vi "TVS Test.vi"(8 "error in (no error)":errorcluster, 10 "Message IN":string) -> (0 "error out":errorcluster, 1 "Result (bool)":bool, 2 "Message OUT":string)   [LabVIEW 2022 SP3]
uses:
  <vilib>/DAQmx/write.llb/DAQmx Write (Digital Bool 1Line 1Point).vi
  <vilib>/DAQmx/read.llb/DAQmx Read (Digital Bool 1Line 1Point).vi
  <vilib>/DAQmx/miscellaneous.llb/DAQmx Fill In Error Info.vi
panel:
  out "DAQ Reading":bool
  out "Result (color)":u32(colorbox)
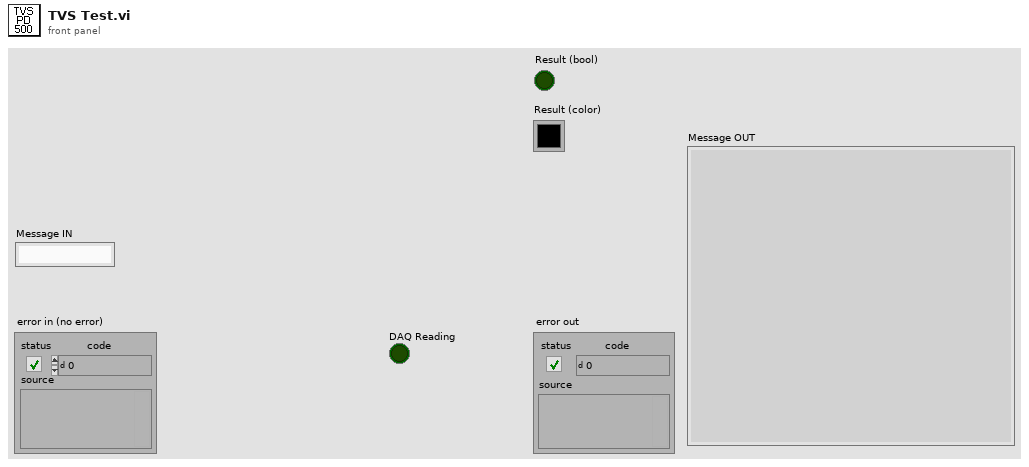
[diagram p1: front panel]
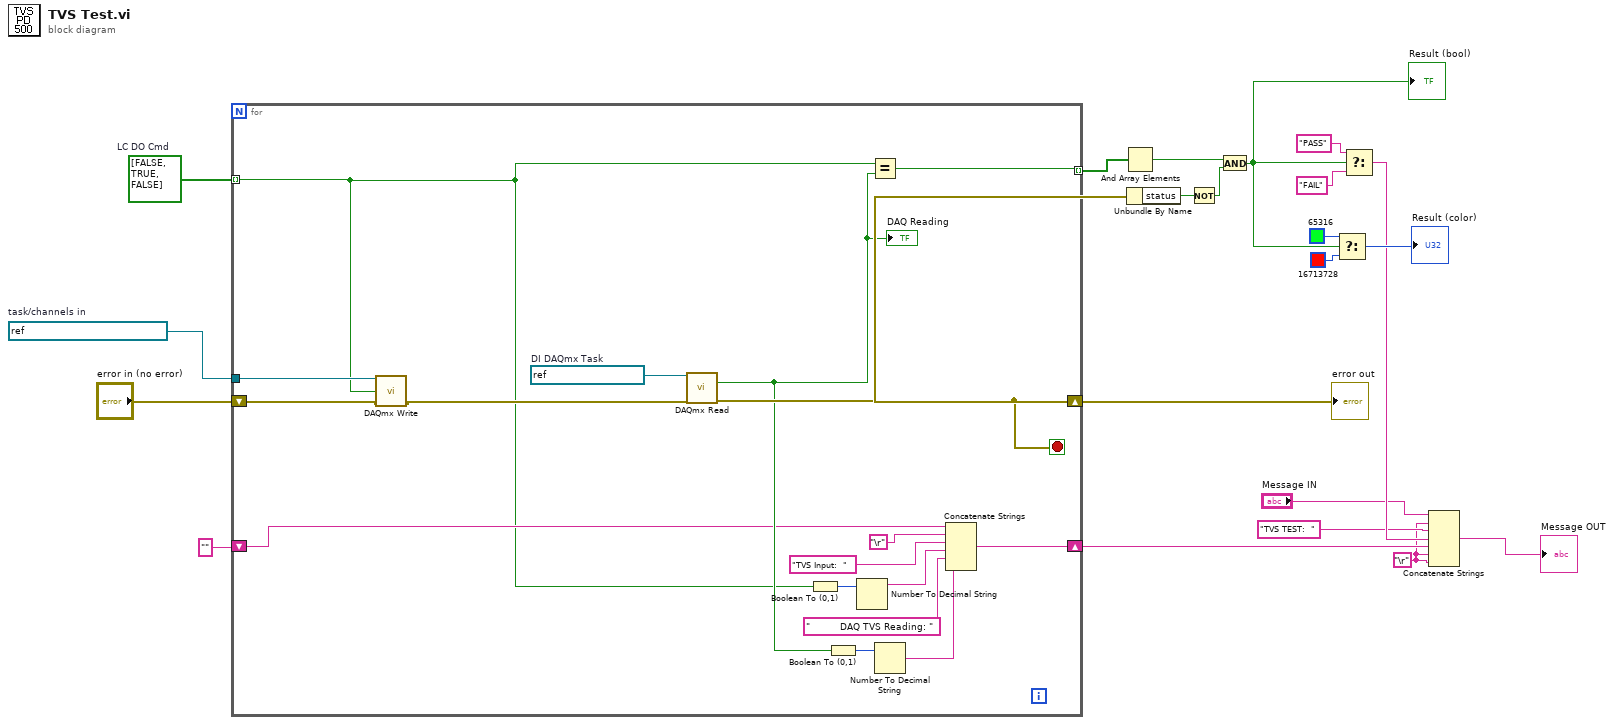
[diagram p0: block diagram]
diagram:
  w1 = refnum<k21> "FTS2_ProgrammingRelay"  # task/channels in
  w2 = bool[] [FALSE, TRUE, FALSE]  # LC DO Cmd
  w4 = "\r"
  n1 = for {
    shift-right: [w37] -> w10
    shift-left: "error in (no error)" -> [w26]
    tunnel: [w22] -> w21 mode=indexing
    shift-right: [w28] -> w9
    shift-left: "" -> [w27]
    tunnel: w2 -> [w23] mode=indexing
    tunnel: w1 -> [w24]
    stop <- w37 stop-if-true
    w38 = refnum<k21> "FTS2_PD500_TVS"  # DI DAQmx Task
    n2 = call-poly <vilib>:"DAQmx Write.vi"("task/channels in"=w24, "data"=w23, "error in"=w26) -> ("error out"=w25:errorcluster)  [unwired: 10 in, 2 out]
    n3 = call-poly <vilib>:"DAQmx Read.vi"("task/channels in"=w38, "error in"=w25) -> ("data"=w29:bool, "error out"=w37:errorcluster)  [unwired: 11 in, 1 out]
    "DAQ Reading" <- w29
    n4 = Boolean To (0,1)(Boolean=w23) -> (0, 1=w31:i16)
    n5 = Boolean To (0,1)(Boolean=w29) -> (0, 1=w30:i16)
    n6 = Number To Decimal String(number=w31) -> (decimal integer string=w34:string)  [unwired: 1 in]
    n7 = Equal?(x=w23, y=w29) -> (x = y?=w22:bool)
    n8 = Number To Decimal String(number=w30) -> (decimal integer string=w36:string)  [unwired: 1 in]
    n9 = Concatenate Strings(w27, "\r", "TVS Input:  ", w34, "          DAQ TVS Reading: ", w36) -> (w28:string)
  }
  "error out" <- w10
  n10 = And Array Elements(Boolean array=w21) -> (logical AND=w11:bool)
  n11 = Unbundle By Name(w10) -> ("status"=w14:bool)
  n12 = Not(x=w14) -> (.not. x?=w13:bool)
  n13 = And(x=w11, y=w13) -> (x .and. y?=w12:bool)
  "Result (bool)" <- w12
  n14 = Select(t=u32 65316 ("Result (color)"), s=w12, f=u32 16713728 ("Result (color)")) -> (s? t:f=→"Result (color)":u32)
  n15 = Select(t="PASS", s=w12, f="FAIL") -> (s? t:f=w7:string)
  n16 = Concatenate Strings("Message IN", w4, "TVS TEST:  ", w7, w9, w4, w4) -> (→"Message OUT":string)
